vi "Write Data.vi"(8 "error in (no error)":errorcluster, 11 "LakeShore370 in":refnum<class "LakeShore370_device.lvclass">) -> (0 "error out":errorcluster, 3 "LakeShore370 out":refnum<class "LakeShore370_device.lvclass">)   [LabVIEW 2015, in "LakeShore370_device.lvclass"]
uses:
  LakeShore370_device.lvclass
  LakeSore370 Front Panel Data.ctl
  LakeShore370 Heater Ranges.ctl
  Neocera/Neocera Set Point Aproach.ctl
  Instrument/Read VISA Resource.vi
  OO Devices/Device/Read Control Panel Loaded.vi
  Instrument/Write VISA Resource.vi
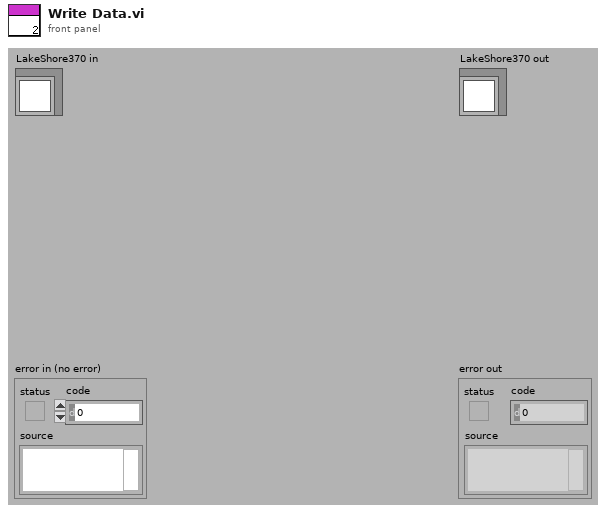
[diagram p1: front panel]
types:
  T1 = typedef "LakeSore370 Front Panel Data.ctl" = cluster{"Channels to scan":i32[], "Scan settling, s":dbl, "Read temperature":bool, "Set point":dbl, "Heater range":T2, "Approach":T3, "Ramp rate, K/min":dbl, "Read heater":bool}
  T2 = typedef "LakeShore370 Heater Ranges.ctl" = enum16{"Off", "31.6uA", "100uA", "316uA", "1mA", "3.16uA", "10mA", "31.6mA", "100mA"}
  T3 = typedef "Neocera Set Point Aproach.ctl" = enum16{"Instant", "Ramp"}
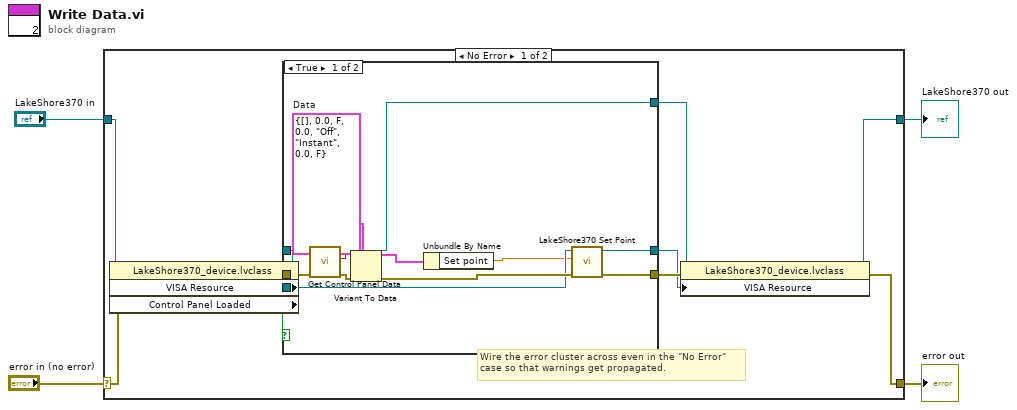
[diagram p0: block diagram]
diagram:
  n1 = case shown="No Error" "error in (no error)" {
    selector: "error in (no error)" -> [w8 w32]
    tunnel: [w7 w32] -> w3
    tunnel: [w6 w31] -> w1
    tunnel: "LakeShore370 in" -> [w9 w31]
    frame No Error {
      # "Wire the error cluster across even in the \"No Error\"\ncase so that warnings get propagated."
      n2 = property class="LakeShore370_device.lvclass"(reference=w9, error in=w8) -> (reference out=w15:refnum<class "LakeShore370_device.lvclass">, error out=w12:errorcluster, "VISA Resource"=w5:refnum<visa-resource-name>, "Control Panel Loaded"=w10:bool)
      n3 = case shown="True" w10 {
        tunnel: w15 -> [w25 w30]
        tunnel: [w24 w30] -> w14
        tunnel: [w19 w28] -> w13
        tunnel: w12 -> [w23 w28]
        tunnel: [w18 w29] -> w11
        tunnel: w5 -> [w17 w29]
        frame True {
          w27 = T1 {"Channels to scan"=[], "Scan settling, s"=0.0, "Read temperature"=FALSE, "Set point"=0.0, "Heater range"=enum."Off", "Approach"=enum."Instant", "Ramp rate, K/min"=0.0, "Read heater"=FALSE}  # Data
          n4 = call-dynamic "Get Control Panel Data.vi"("error in (no error)"=w23, "Device in"=w25) -> ("error out"=w22:errorcluster, "Data"=w21:variant, "Device out"=w24:refnum<class "LakeShore370_device.lvclass">)  [unwired: 7 in]
          n5 = Variant To Data(error in=w22, type=w27, Variant=w21) -> (data=w26:T1, error out=w20:errorcluster)
          n6 = Unbundle By Name(w26) -> ("Set point"=w16:dbl)
          n7 = call "LakeShore370 Set Point.vi"("error in (no error)"=w20, "Set Point"=w16, "VISA resource name"=w17) -> ("error out"=w19:errorcluster, "VISA resource name out"=w18:refnum<visa-resource-name>)  [unwired: 7 in]
        }
        frame False {
        }
      }
      n8 = property class="LakeShore370_device.lvclass"(reference=w14, error in=w13, "VISA Resource"=w11) -> (reference out=w6:refnum<class "LakeShore370_device.lvclass">, error out=w7:errorcluster)
    }
    frame Error {
    }
  }
  "error out" <- w3
  "LakeShore370 out" <- w1
